vi "5p1_HW_Task2_gamagetd.vi"() -> ()   [LabVIEW 2016]
panel:
  out "Result":string
  in  "Second Derivative f'' (x)":dbl
  in  "First Derivative f'(x)":dbl
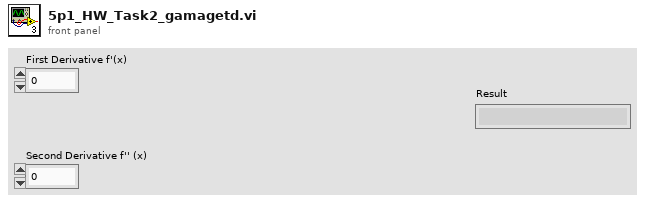
[diagram p1: front panel]
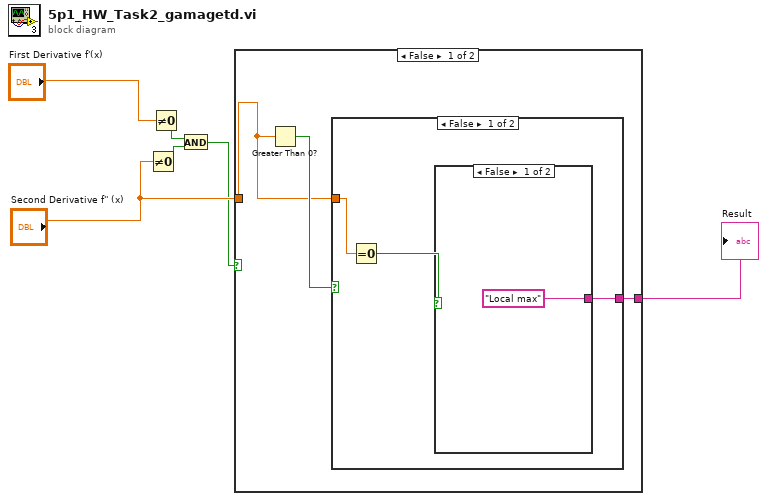
[diagram p0: block diagram]
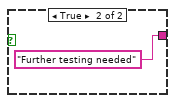
[diagram p2: hidden frame]
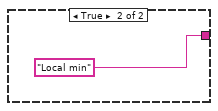
[diagram p3: hidden frame]
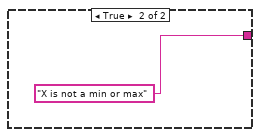
[diagram p4: hidden frame]
diagram:
  n1 = Not Equal To 0?(x="Second Derivative f'' (x)") -> (x != 0?=w3:bool)
  n2 = Not Equal To 0?(x="First Derivative f'(x)") -> (x != 0?=w4:bool)
  n3 = And(x=w4, y=w3) -> (x .and. y?=w1:bool)
  n4 = case shown="False" w1 {
    tunnel: "Second Derivative f'' (x)" -> [w8 _]
    tunnel: [w7 "X is not a min or max"] -> w2
    frame False {
      n5 = Greater Than 0?(x=w8) -> (x > 0?=w9:bool)
      n6 = case shown="False" w9 {
        tunnel: w8 -> [w12 _]
        tunnel: [w11 "Local min"] -> w7
        frame False {
          n7 = Equal To 0?(x=w12) -> (x = 0?=w10:bool)
          n8 = case shown="False" w10 {
            tunnel: ["Local max" "Further testing needed"] -> w11
            frame False {
            }
            frame True {
            }
          }
        }
        frame True {
        }
      }
    }
    frame True {
    }
  }
  "Result" <- w2
